vi "Save data to SQL.vi"(8 "error in (no error)":errorcluster, 11 "data in":string) -> (2 "Error out sql":errorcluster, 7 "Data":string[][](array[string]))   [LabVIEW 2020]
panel:
  out "time":string
  out "angle":string
  out "password":string
  out "address":string
  out "name":string
  out "Id":string
  out "phone":string
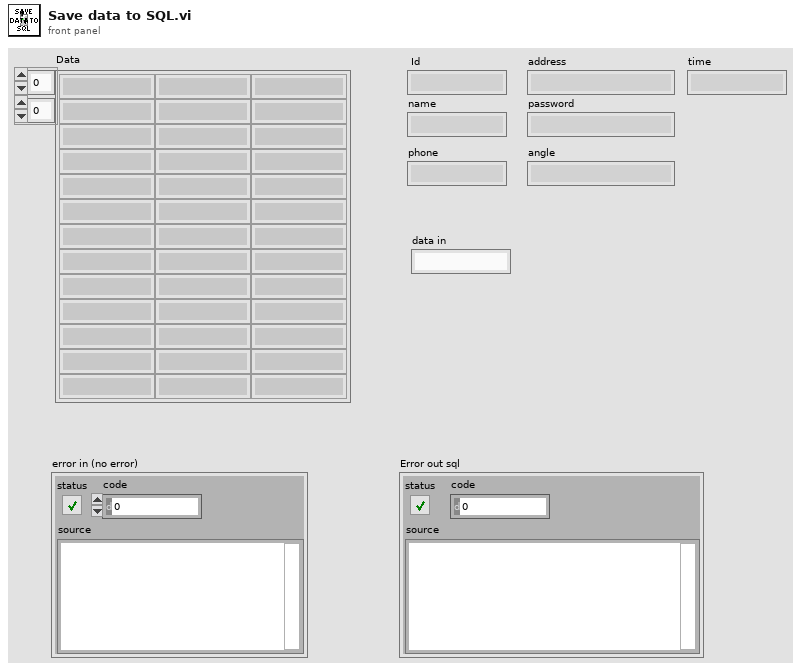
[diagram p1: front panel]
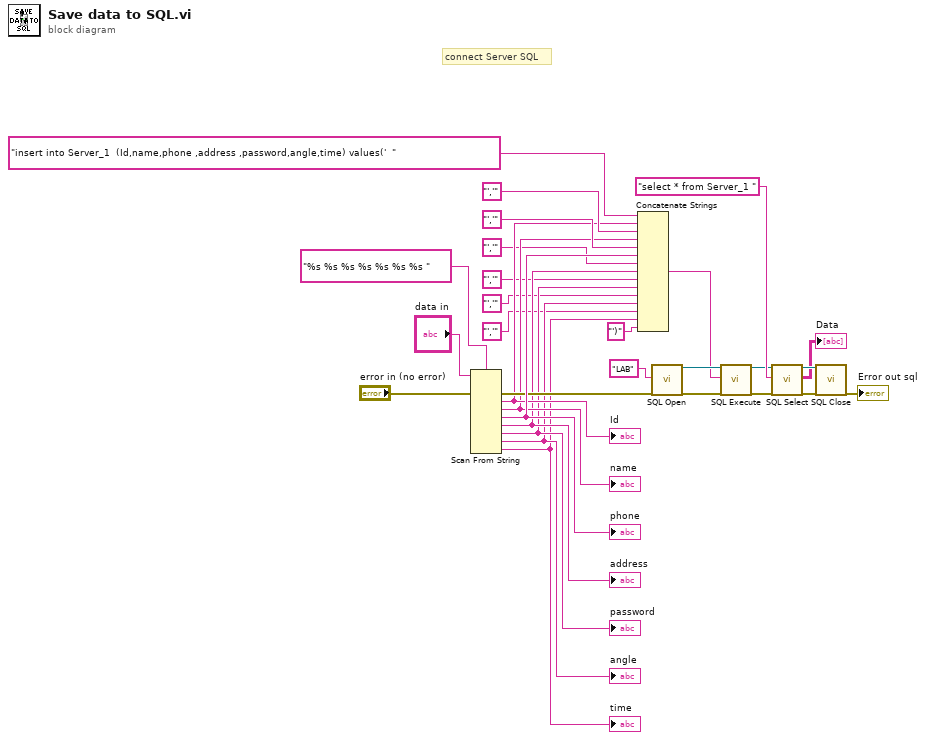
[diagram p0: block diagram]
diagram:
  # "connect Server SQL"
  n1 = Scan From String(format string="%s %s %s %s %s %s %s ", input string="data in", error in="error in (no error)") -> (error out=w12:errorcluster, output 1=w11:string, output 2=w10:string, output 3=w14:string, output 4=w8:string, output 5=w7:string, output 6=w6:string, output 7=w5:string)  [unwired: 8 in, 2 out]
  "phone" <- w14
  "Id" <- w11
  "name" <- w10
  "address" <- w8
  "password" <- w7
  "angle" <- w6
  "time" <- w5
  n2 = Concatenate Strings("insert into Server_1  (Id,name,phone ,address ,password,angle,time) values('  " ("SQL Query"), w11, "','" ("string"), w10, "','" ("string"), w14, "','" ("string"), w8, "','" ("string"), w7, "','" ("string"), w6, "','" ("string"), w5, "')" ("string")) -> (w17:string)
  n3 = call <vilib>:"SQL Open.vi"("ConnectionString In"="LAB", "Error in (no error)"=w12) -> ("Connection Out"=w20:refnum<k7>, "Error out"=w19:errorcluster)  [unwired: 16 in]
  n4 = call <vilib>:"SQL Execute.vi"("Connection In"=w20, "SQL Query"=w17, "Error in (no error)"=w19) -> ("Connection Out"=w18:refnum<k7>, "Error out"=w13:errorcluster)  [unwired: 15 in]
  n5 = call <vilib>:"SQL Select.vi"("Connection In"=w18, "SQL Query"="select * from Server_1 ", "Error in (no error)"=w13) -> ("Connection Out"=w23:refnum<k7>, "Data"=→"Data":string[][], "Error out"=w22:errorcluster)  [unwired: 14 in]
  n6 = call <vilib>:"SQL Close.vi"("Connection In"=w23, "Error in (no error)"=w22) -> ("Error out"=→"Error out sql":errorcluster)  [unwired: 17 in]
